vi "pumonarytesting_auto_attempt5.vi"() -> ()   [LabVIEW 2014]
uses:
  <vilib>/vision/NI_Vision_Development_Module.lvlib
  <instrlib>/KD Scientific 2XX Series/KD Scientific 2XX Series.lvlib
panel:
  in  "Start Pressure":i32=20
  in  "Number of Cycles":i32
  in  "Min Pressure":dbl
  in  "Max Pressure":dbl
  out "Status":T1
  in  "stop 2":bool
  out "Delivered Volume":dbl
  out "Units":string
  in  "Baud Rate (9600)":u32(ring)=9600 items=["300"=300, "1200"=1200, "2400"=2400, "4800"=4800, "9600"=9600]
  in  "Withdrawal Settings":T2={"Flow Rate (5)"=5.0, "Volume (10)"=10.0, "Volume Units (ml)"=enum."milliliters (ml)", "Rate Units (ml/min.)"=enum."milliliters per minute (ml/min.)"} {"Volume (10)" format="%#.3g"}
  in  "Diameter (8.75 mm)":dbl=8.75
  in  "Infusion Settings":T2={"Flow Rate (5)"=5.0, "Volume (10)"=10.0, "Volume Units (ml)"=enum."milliliters (ml)", "Rate Units (ml/min.)"=enum."milliliters per minute (ml/min.)"}
  in  "Address (0)":i32 format="%0.0f"
  in  "error in (no error)":errorcluster
  in  "VISA resource name":refnum<visa-resource-name>="COM1"
  in  "stop 4":bool
  in  "stop":bool
  out "Image":T3(plugin-control)
  out "Particle Measurements (Pixels) (Particle Analysis 1)":dbl[][](array[numeric]) format="%.2f"
  out "subarray":dbl[](array[numeric])
  out "The diameter":dbl[](array[numeric])
  in  "stop (F)":bool
  out "Data from Transducer":dynamicdata(graph) caption="Voltage from Transducer V"
  out "Voltage from pressure transducer":dbl[](array[numeric])
  out "Pressure mm Hg":dbl[](graph)
  in  "Calibration factor":dbl[](array[numeric])
  in  "Zero Error":dbl[](array[numeric])
  out "pressure mm Hg":dbl[](array[numeric])
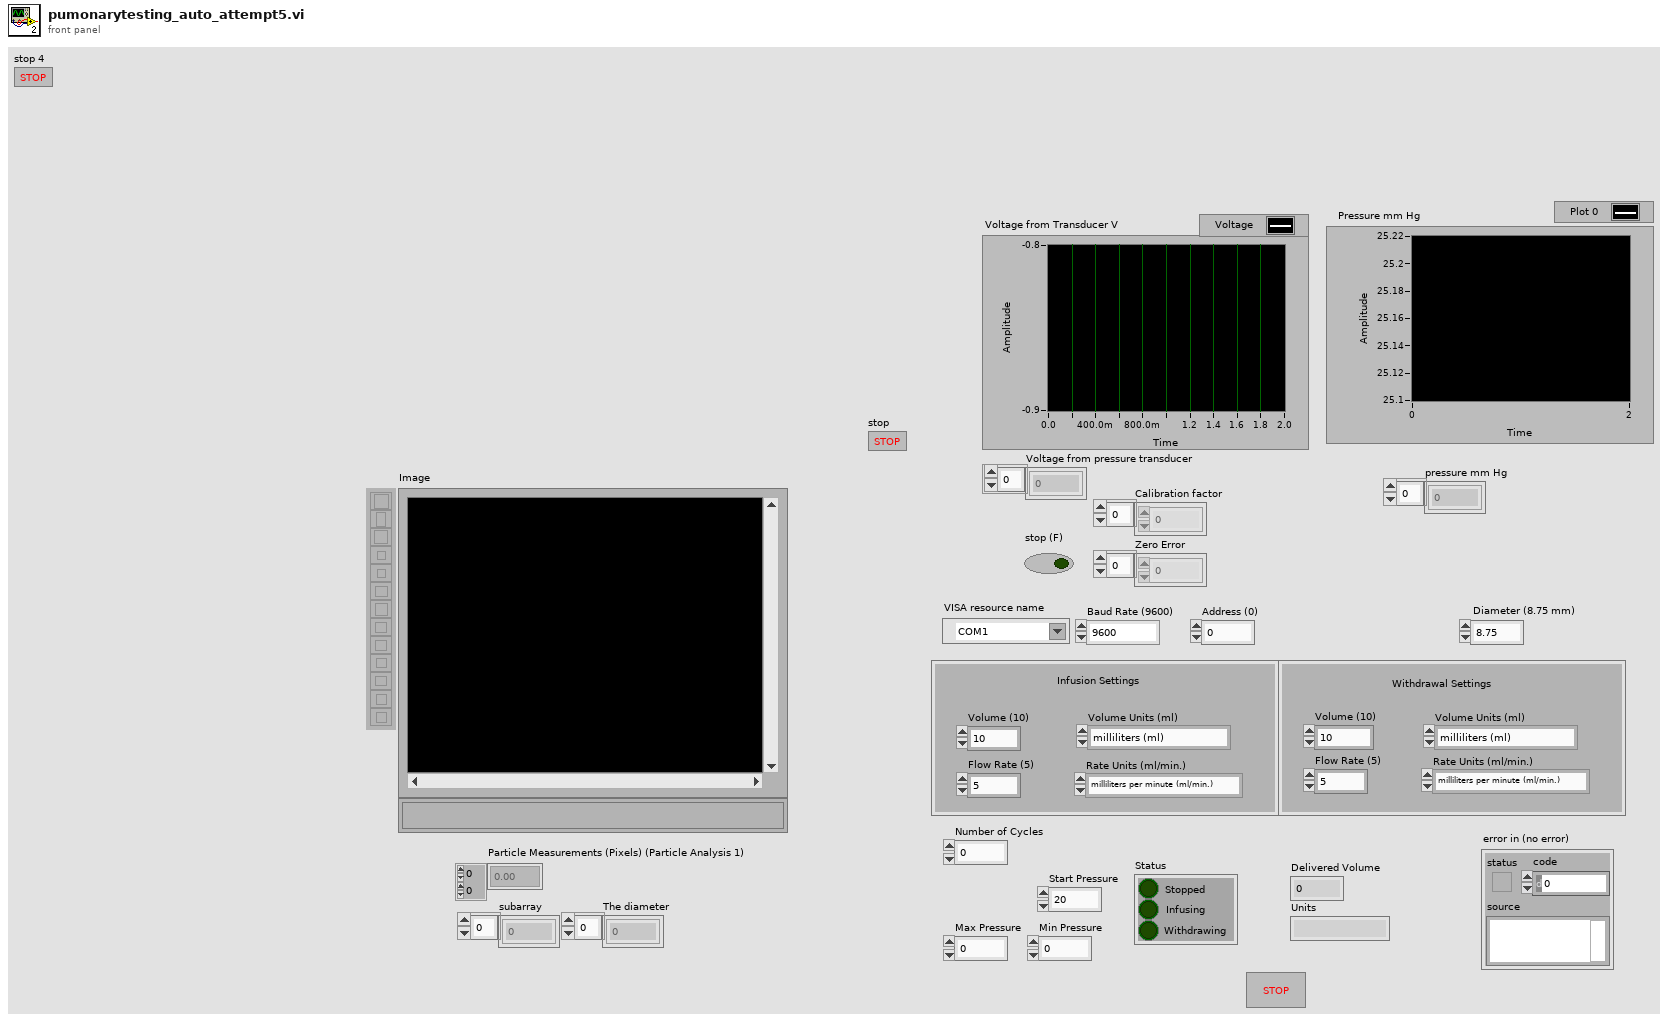
[diagram p1: front panel]
types:
  T1 = cluster{"Stopped":bool, "Infusing":bool, "Withdrawing":bool}
  T2 = cluster{"Flow Rate (5)":dbl, "Volume (10)":dbl, "Volume Units (ml)":enum16{"milliliters (ml)", "microliters (ul)"}, "Rate Units (ml/min.)":enum16{"milliliters per minute (ml/min.)", "milliliters per hour (ml/hr.)", "microliters per minute (ul/min.)", "microliters per hour (ul/hr.)"}}
  T3 = typedef "IMAQ Image.ctl" = refnum<image>
  T4 = typedef "Board Id" = u8
  T5 = typedef "ROI Descriptor" = cluster{"Global Rectangle":i32[], "Contours":cluster{"ID":enum32{"External", "Internal"}, "Type":u32, "Coordinates":i32[]}[]}
  T6 = enum16{"milliliters per minute (ml/min.)", "milliliters per hour (ml/hr.)", "microliters per minute (ul/min.)", "microliters per hour (ul/hr.)"}
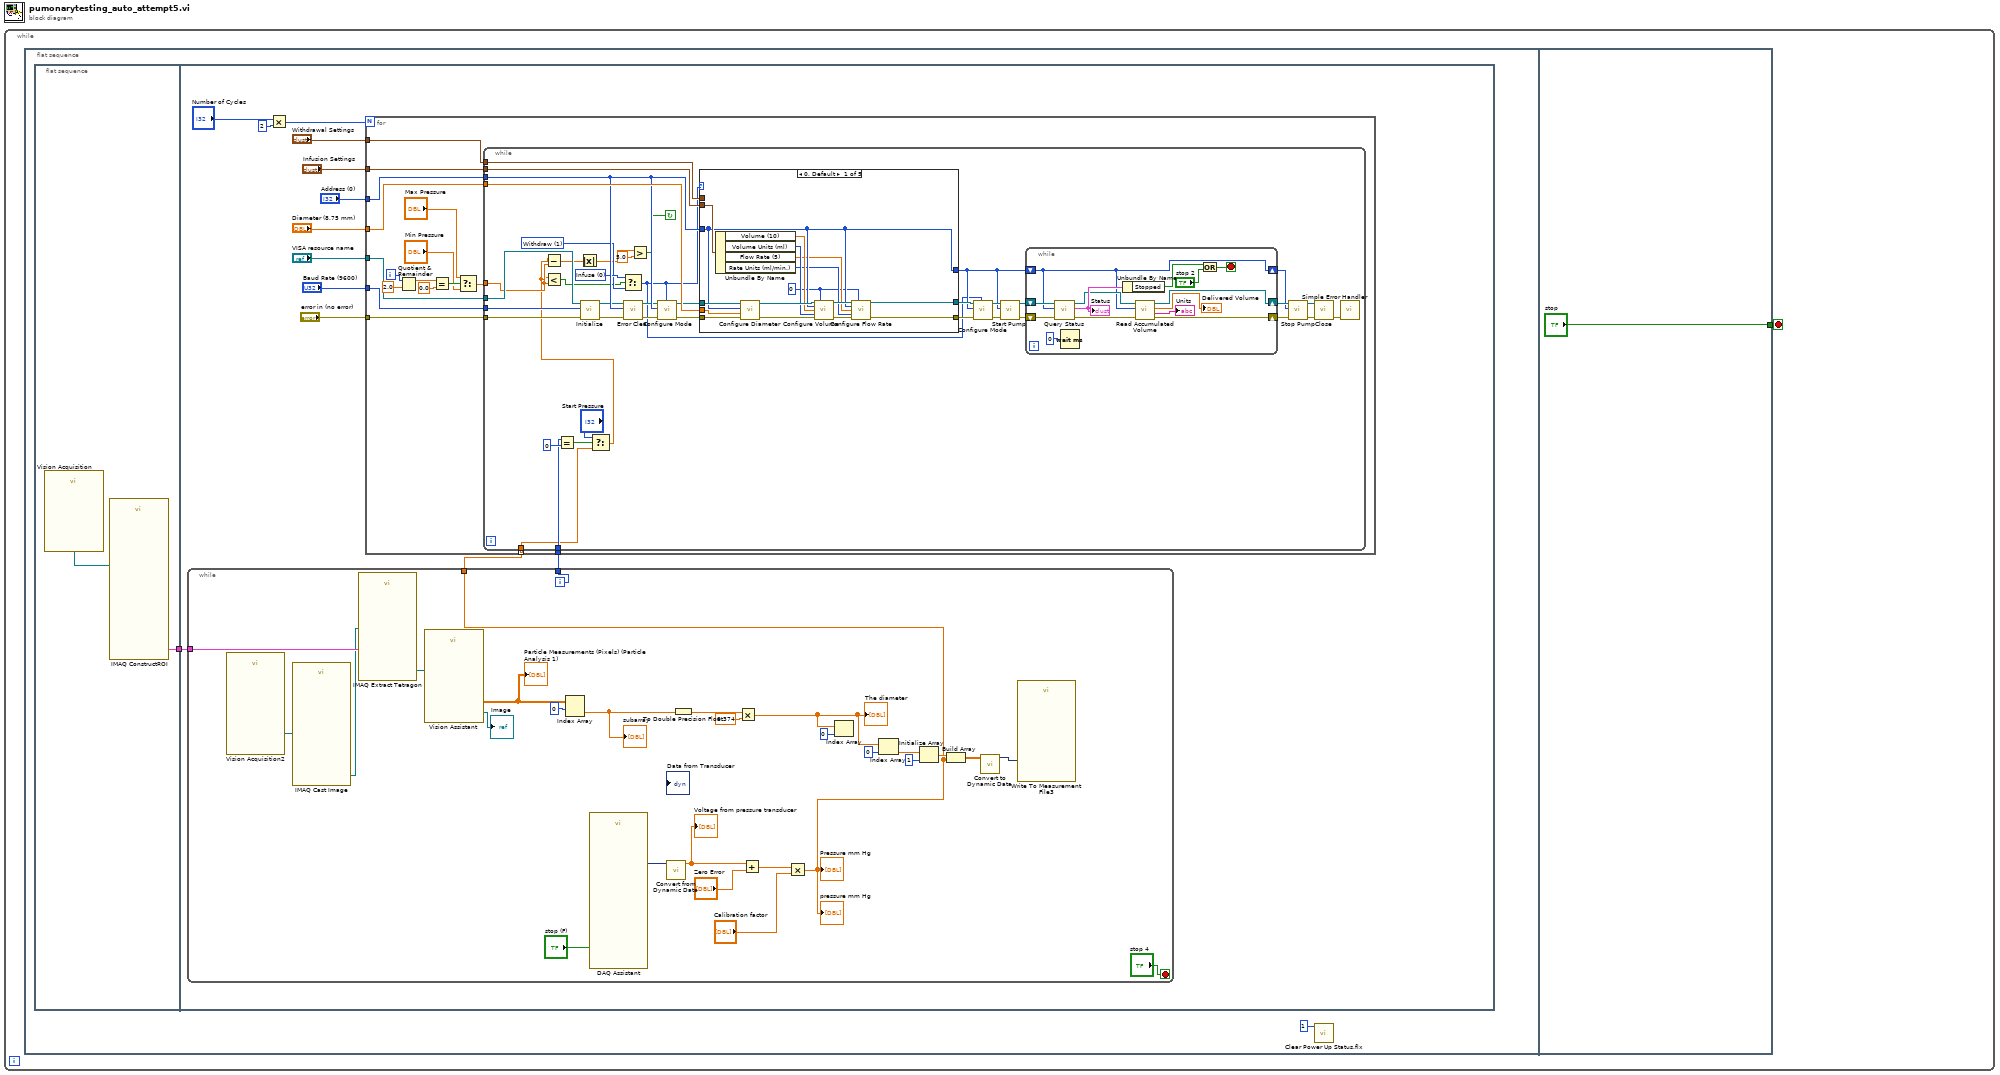
[diagram p0: block diagram]
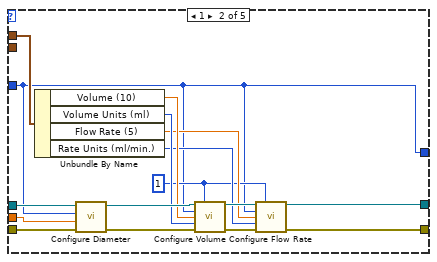
[diagram p2: hidden frame]
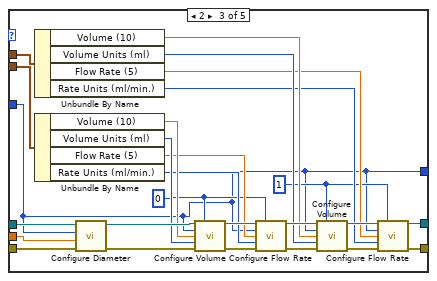
[diagram p3: hidden frame]
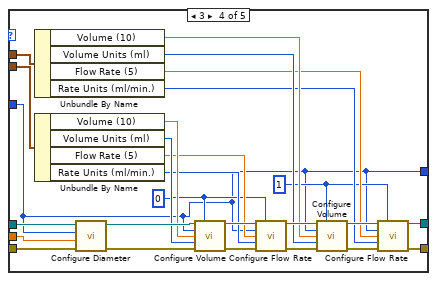
[diagram p4: hidden frame]
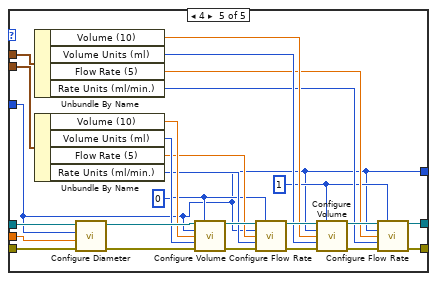
[diagram p5: hidden frame]
diagram:
  n1 = while {
    stop <- w1 stop-if-true
    n2 = flat-sequence {
      tunnel: ["stop"] -> w1
      frame #0 {
        n3 = flat-sequence {
          tunnel: [w4] -> w3
          tunnel: w3 -> [w18]
          frame #0 {
            n4 = call "Vision Acquisition"() -> ("Image Out"=w5:T3)  [unwired: 26 in, 1 out]
            n5 = call "IMAQ ConstructROI"("Image"=w5) -> ("ROI Descriptor Out"=w4:T5)  [unwired: 7 in, 3 out]
          }
          frame #1 {
            n6 = while {
              tunnel: w18 -> [w227]
              tunnel: [w202] -> w7
              tunnel: [w201] -> w6
              i -> [w201]
              stop <- "stop 4" stop-if-true
              n7 = call "Vision Acquisition2"() -> ("Image Out"=w217:T3)  [unwired: 25 in, 2 out]
              n8 = call "IMAQ Cast Image"("Image Src"=w217) -> ("Image Dst Out"=w224:T3)  [unwired: 9 in, 1 out]
              n9 = call-poly "IMAQ Extract Tetragon"("ROI Descriptor"=w227, "Image Src"=w224) -> ("Image Dst Out"=w225:T3)  [unwired: 8 in, 1 out]
              n10 = call "Vision Assistant"("Image In"=w225) -> ("Image Out"=→"Image":T3, "Particle Measurements (Pixels) (Particle Analysis 1)"=w223:dbl[][])  [unwired: 23 in, 2 out]
              "Particle Measurements (Pixels) (Particle Analysis 1)" <- w223
              n11 = Index Array(array=w223, index (row)=0) -> (element=w221:dbl[])  [unwired: 1 in]
              "subarray" <- w221
              n12 = call "DAQ Assistant"("stop (F)"="stop (F)") -> ("data"=w208:dynamicdata)  [unwired: 15 in, 3 out]
              n13 = call "Convert from Dynamic Data"("Dynamic Data Type"=w208) -> ("Array"=w205:dbl[])  [unwired: 3 in]
              "Voltage from pressure transducer" <- w205
              n14 = To Double Precision Float(number=w221) -> (double precision float=w220:dbl[])
              n15 = Multiply(x=w220, y=0.374) -> (x*y=w214:dbl[])
              "The diameter" <- w214
              n16 = Add(x=w205, y="Zero Error") -> (x+y=w207:dbl[])
              n17 = Multiply(x=w207, y="Calibration factor") -> (x*y=w202:dbl[])
              "Pressure mm Hg" <- w202
              "pressure mm Hg" <- w202
              n18 = Index Array(array=w214, index=0) -> ()  [unwired: 1 out]
              n19 = Index Array(array=w214, index=0) -> (element=w213:dbl)
              n20 = Initialize Array(w213, 1 ("dimension size")) -> (w211:dbl[])
              n21 = Build Array(w211, w202) -> (w210:dbl[][])
              n22 = call "Convert to Dynamic Data"("2D Array"=w210) -> ("Dynamic Data Type"=w209:dynamicdata)  [unwired: 3 in]
              n23 = call "Write To Measurement File3"("Signals"=w209) -> ()  [unwired: 16 in, 3 out]
            }
            n24 = Multiply(x="Number of Cycles", y=2) -> (x*y=w17:i32)
            n25 = for {
              N: w17 -> [_]
              tunnel: "VISA resource name" -> [w35]
              tunnel: "error in (no error)" -> [w34]
              tunnel: "Infusion Settings" -> [w33]
              tunnel: "Withdrawal Settings" -> [w32]
              tunnel: "Diameter (8.75 mm)" -> [w31]
              tunnel: "Baud Rate (9600)" -> [w30]
              tunnel: "Address (0)" -> [w29]
              tunnel: w7 -> [w20] mode=indexing
              tunnel: w6 -> [w19]
              i -> [w27]
              n26 = Quotient & Remainder(x=w27, y=2.0) -> (x-y*floor(x/y)=w25:dbl)  [unwired: 1 out]
              n27 = Equal?(x=w25, y=0.0) -> (x = y?=w24:bool)
              n28 = Select(t="Max Pressure", s=w24, f="Min Pressure") -> (s? t:f=w21:dbl)
              n29 = while {
                tunnel: w35 -> [w76]
                tunnel: w34 -> [w75]
                tunnel: w33 -> [w74]
                tunnel: w32 -> [w73]
                tunnel: w31 -> [w72]
                tunnel: w30 -> [w71]
                tunnel: w29 -> [w70]
                tunnel: w21 -> [w47]
                tunnel: w20 -> [w37]
                tunnel: w19 -> [w39]
                stop <- w42 continue-if-true
                w49 = u16 1 items=["Withdraw"=1]
                w50 = u16 0 items=["Infuse"] ("Mode (infuse)")
                n30 = Equal?(x=w39, y=0) -> (x = y?=w40:bool)
                n31 = call <instrlib>:"Initialize.vi"("error in (no error)"=w75, "Baud Rate (9600)"=w71, "VISA resource name"=w76) -> ("error out"=w52:errorcluster, "VISA resource name out"=w51:refnum<visa-resource-name>)  [unwired: 7 in]
                n32 = Select(t="Start Pressure", s=w40, f=w37) -> (s? t:f=w36:dbl)
                n33 = Subtract(x=w36, y=w47) -> (x-y=w46:dbl)
                n34 = Less?(x=w36, y=w47) -> (x < y?=w43:bool)
                n35 = Absolute Value(x=w46) -> (abs(x)=w45:dbl)
                n36 = Select(t=w50, s=w43, f=w49) -> (s? t:f=w48:u16)
                n37 = call <instrlib>:"Error Clear.vi"("error in (no error)"=w52, "Address (0)"=w70, "VISA resource name"=w51) -> ("error out"=w53:errorcluster, "VISA resource name out"=w54:refnum<visa-resource-name>)  [unwired: 6 in, 1 out]
                n38 = Greater?(x=w45, y=5.0) -> (0:w42:bool)
                n39 = call <instrlib>:"Configure Mode.vi"("Mode (infuse)"=w48, "error in (no error)"=w53, "Address (0)"=w70, "VISA resource name"=w54) -> ("error out"=w56:errorcluster, "VISA resource name out"=w55:refnum<visa-resource-name>)  [unwired: 6 in]
                n40 = case shown="0, Default" w48 {
                  tunnel: w74 -> [w86 _ w134 w160 w186]
                  tunnel: w73 -> [_ w108 w133 w159 w185]
                  tunnel: w55 -> [w92 w107 w132 w158 w184]
                  tunnel: w56 -> [w91 w103 w131 w157 w183]
                  tunnel: w72 -> [w85 w99 w114 w140 w166]
                  tunnel: [w84 w93 w109 w135 w161] -> w57
                  tunnel: w70 -> [w84 w93 w109 w135 w161]
                  tunnel: [w79 w104 w111 w137 w163] -> w61
                  tunnel: [w78 w100 w110 w136 w162] -> w60
                  frame 0, Default {
                    w77 = 0
                    n41 = Unbundle By Name(w86) -> ("Volume (10)"=w83:dbl, "Volume Units (ml)"=w82:enum16{"milliliters (ml)", "microliters (ul)"}, "Flow Rate (5)"=w81:dbl, "Rate Units (ml/min.)"=w80:T6)
                    n42 = call <instrlib>:"Configure Diameter.vi"("error in (no error)"=w91, "Diameter (8.75 mm)"=w85, "Address (0)"=w84, "VISA resource name"=w92) -> ("error out"=w89:errorcluster, "VISA resource name out"=w90:refnum<visa-resource-name>)  [unwired: 6 in]
                    n43 = call <instrlib>:"Configure Volume.vi"("VISA resource name"=w90, "Mode (infuse)"=w77, "Address (0)"=w84, "Volume (100)"=w83, "Units (0: milliliters)"=w82, "error in (no error)"=w89) -> ("VISA resource name out"=w88:refnum<visa-resource-name>, "error out"=w87:errorcluster)  [unwired: 8 in]
                    n44 = call <instrlib>:"Configure Flow Rate.vi"("VISA resource name"=w88, "Mode (infuse)"=w77, "Address (0)"=w84, "Flow Rate (5)"=w81, "Units (0: milliliters per minute)"=w80, "error in (no error)"=w87) -> ("VISA resource name out"=w79:refnum<visa-resource-name>, "error out"=w78:errorcluster)  [unwired: 8 in]
                  }
                  frame 1 {
                    w94 = 1
                    n45 = Unbundle By Name(w108) -> ("Volume (10)"=w98:dbl, "Volume Units (ml)"=w97:enum16{"milliliters (ml)", "microliters (ul)"}, "Flow Rate (5)"=w96:dbl, "Rate Units (ml/min.)"=w95:T6)
                    n46 = call <instrlib>:"Configure Diameter.vi"("error in (no error)"=w103, "Diameter (8.75 mm)"=w99, "Address (0)"=w93, "VISA resource name"=w107) -> ("error out"=w102:errorcluster, "VISA resource name out"=w106:refnum<visa-resource-name>)  [unwired: 6 in]
                    n47 = call <instrlib>:"Configure Volume.vi"("VISA resource name"=w106, "Mode (infuse)"=w94, "Address (0)"=w93, "Volume (100)"=w98, "Units (0: milliliters)"=w97, "error in (no error)"=w102) -> ("VISA resource name out"=w105:refnum<visa-resource-name>, "error out"=w101:errorcluster)  [unwired: 8 in]
                    n48 = call <instrlib>:"Configure Flow Rate.vi"("VISA resource name"=w105, "Mode (infuse)"=w94, "Address (0)"=w93, "Flow Rate (5)"=w96, "Units (0: milliliters per minute)"=w95, "error in (no error)"=w101) -> ("VISA resource name out"=w104:refnum<visa-resource-name>, "error out"=w100:errorcluster)  [unwired: 8 in]
                  }
                  frame 2 {
                    w112 = 1
                    w113 = 0
                    n49 = Unbundle By Name(w133) -> ("Volume (10)"=w118:dbl, "Volume Units (ml)"=w117:enum16{"milliliters (ml)", "microliters (ul)"}, "Flow Rate (5)"=w116:dbl, "Rate Units (ml/min.)"=w115:T6)
                    n50 = Unbundle By Name(w134) -> ("Volume (10)"=w122:dbl, "Volume Units (ml)"=w121:enum16{"milliliters (ml)", "microliters (ul)"}, "Flow Rate (5)"=w120:dbl, "Rate Units (ml/min.)"=w119:T6)
                    n51 = call <instrlib>:"Configure Diameter.vi"("error in (no error)"=w131, "Diameter (8.75 mm)"=w114, "Address (0)"=w109, "VISA resource name"=w132) -> ("error out"=w126:errorcluster, "VISA resource name out"=w130:refnum<visa-resource-name>)  [unwired: 6 in]
                    n52 = call <instrlib>:"Configure Volume.vi"("VISA resource name"=w130, "Mode (infuse)"=w113, "Address (0)"=w109, "Volume (100)"=w122, "Units (0: milliliters)"=w121, "error in (no error)"=w126) -> ("VISA resource name out"=w129:refnum<visa-resource-name>, "error out"=w125:errorcluster)  [unwired: 8 in]
                    n53 = call <instrlib>:"Configure Flow Rate.vi"("VISA resource name"=w129, "Mode (infuse)"=w113, "Address (0)"=w109, "Flow Rate (5)"=w120, "Units (0: milliliters per minute)"=w119, "error in (no error)"=w125) -> ("VISA resource name out"=w128:refnum<visa-resource-name>, "error out"=w124:errorcluster)  [unwired: 8 in]
                    n54 = call <instrlib>:"Configure Volume.vi"("VISA resource name"=w128, "Mode (infuse)"=w112, "Address (0)"=w109, "Volume (100)"=w118, "Units (0: milliliters)"=w117, "error in (no error)"=w124) -> ("VISA resource name out"=w127:refnum<visa-resource-name>, "error out"=w123:errorcluster)  [unwired: 8 in]
                    n55 = call <instrlib>:"Configure Flow Rate.vi"("VISA resource name"=w127, "Mode (infuse)"=w112, "Address (0)"=w109, "Flow Rate (5)"=w116, "Units (0: milliliters per minute)"=w115, "error in (no error)"=w123) -> ("VISA resource name out"=w111:refnum<visa-resource-name>, "error out"=w110:errorcluster)  [unwired: 8 in]
                  }
                  frame 3 {
                    w138 = 1
                    w139 = 0
                    n56 = Unbundle By Name(w159) -> ("Volume (10)"=w144:dbl, "Volume Units (ml)"=w143:enum16{"milliliters (ml)", "microliters (ul)"}, "Flow Rate (5)"=w142:dbl, "Rate Units (ml/min.)"=w141:T6)
                    n57 = Unbundle By Name(w160) -> ("Volume (10)"=w148:dbl, "Volume Units (ml)"=w147:enum16{"milliliters (ml)", "microliters (ul)"}, "Flow Rate (5)"=w146:dbl, "Rate Units (ml/min.)"=w145:T6)
                    n58 = call <instrlib>:"Configure Diameter.vi"("error in (no error)"=w157, "Diameter (8.75 mm)"=w140, "Address (0)"=w135, "VISA resource name"=w158) -> ("error out"=w152:errorcluster, "VISA resource name out"=w156:refnum<visa-resource-name>)  [unwired: 6 in]
                    n59 = call <instrlib>:"Configure Volume.vi"("VISA resource name"=w156, "Mode (infuse)"=w139, "Address (0)"=w135, "Volume (100)"=w148, "Units (0: milliliters)"=w147, "error in (no error)"=w152) -> ("VISA resource name out"=w155:refnum<visa-resource-name>, "error out"=w151:errorcluster)  [unwired: 8 in]
                    n60 = call <instrlib>:"Configure Flow Rate.vi"("VISA resource name"=w155, "Mode (infuse)"=w139, "Address (0)"=w135, "Flow Rate (5)"=w146, "Units (0: milliliters per minute)"=w145, "error in (no error)"=w151) -> ("VISA resource name out"=w154:refnum<visa-resource-name>, "error out"=w150:errorcluster)  [unwired: 8 in]
                    n61 = call <instrlib>:"Configure Volume.vi"("VISA resource name"=w154, "Mode (infuse)"=w138, "Address (0)"=w135, "Volume (100)"=w144, "Units (0: milliliters)"=w143, "error in (no error)"=w150) -> ("VISA resource name out"=w153:refnum<visa-resource-name>, "error out"=w149:errorcluster)  [unwired: 8 in]
                    n62 = call <instrlib>:"Configure Flow Rate.vi"("VISA resource name"=w153, "Mode (infuse)"=w138, "Address (0)"=w135, "Flow Rate (5)"=w142, "Units (0: milliliters per minute)"=w141, "error in (no error)"=w149) -> ("VISA resource name out"=w137:refnum<visa-resource-name>, "error out"=w136:errorcluster)  [unwired: 8 in]
                  }
                  frame 4 {
                    w164 = 1
                    w165 = 0
                    n63 = Unbundle By Name(w185) -> ("Volume (10)"=w170:dbl, "Volume Units (ml)"=w169:enum16{"milliliters (ml)", "microliters (ul)"}, "Flow Rate (5)"=w168:dbl, "Rate Units (ml/min.)"=w167:T6)
                    n64 = Unbundle By Name(w186) -> ("Volume (10)"=w174:dbl, "Volume Units (ml)"=w173:enum16{"milliliters (ml)", "microliters (ul)"}, "Flow Rate (5)"=w172:dbl, "Rate Units (ml/min.)"=w171:T6)
                    n65 = call <instrlib>:"Configure Diameter.vi"("error in (no error)"=w183, "Diameter (8.75 mm)"=w166, "Address (0)"=w161, "VISA resource name"=w184) -> ("error out"=w178:errorcluster, "VISA resource name out"=w182:refnum<visa-resource-name>)  [unwired: 6 in]
                    n66 = call <instrlib>:"Configure Volume.vi"("VISA resource name"=w182, "Mode (infuse)"=w165, "Address (0)"=w161, "Volume (100)"=w174, "Units (0: milliliters)"=w173, "error in (no error)"=w178) -> ("VISA resource name out"=w181:refnum<visa-resource-name>, "error out"=w177:errorcluster)  [unwired: 8 in]
                    n67 = call <instrlib>:"Configure Flow Rate.vi"("VISA resource name"=w181, "Mode (infuse)"=w165, "Address (0)"=w161, "Flow Rate (5)"=w172, "Units (0: milliliters per minute)"=w171, "error in (no error)"=w177) -> ("VISA resource name out"=w180:refnum<visa-resource-name>, "error out"=w176:errorcluster)  [unwired: 8 in]
                    n68 = call <instrlib>:"Configure Volume.vi"("VISA resource name"=w180, "Mode (infuse)"=w164, "Address (0)"=w161, "Volume (100)"=w170, "Units (0: milliliters)"=w169, "error in (no error)"=w176) -> ("VISA resource name out"=w179:refnum<visa-resource-name>, "error out"=w175:errorcluster)  [unwired: 8 in]
                    n69 = call <instrlib>:"Configure Flow Rate.vi"("VISA resource name"=w179, "Mode (infuse)"=w164, "Address (0)"=w161, "Flow Rate (5)"=w168, "Units (0: milliliters per minute)"=w167, "error in (no error)"=w175) -> ("VISA resource name out"=w163:refnum<visa-resource-name>, "error out"=w162:errorcluster)  [unwired: 8 in]
                  }
                }
                n70 = call <instrlib>:"Configure Mode.vi"("Mode (infuse)"=w48, "error in (no error)"=w60, "Address (0)"=w57, "VISA resource name"=w61) -> ("error out"=w58:errorcluster, "VISA resource name out"=w59:refnum<visa-resource-name>)  [unwired: 6 in]
                n71 = call <instrlib>:"Start Pump.vi"("error in (no error)"=w58, "Address (0)"=w57, "VISA resource name"=w59) -> ("error out"=w68:errorcluster, "VISA resource name out"=w69:refnum<visa-resource-name>)  [unwired: 7 in]
                n72 = while {
                  shift-right: [w189] -> w65
                  shift-left: w57 -> [w189]
                  shift-right: [w191] -> w67
                  shift-left: w69 -> [w197]
                  shift-right: [w190] -> w66
                  shift-left: w68 -> [w198]
                  stop <- w195 stop-if-true
                  n73 = call <instrlib>:"Query Status.vi"("error in (no error)"=w198, "Address (0)"=w189, "VISA resource name"=w197) -> ("error out"=w200:errorcluster, "Status"=w196:T1, "VISA resource name out"=w192:refnum<visa-resource-name>)  [unwired: 6 in]
                  "Status" <- w196
                  n74 = Wait (ms)(milliseconds to wait=u32 0) -> ()  [unwired: 1 out]
                  n75 = Unbundle By Name(w196) -> ("Stopped"=w194:bool)
                  n76 = call <instrlib>:"Read Accumulated Volume.vi"("error in (no error)"=w200, "Address (0)"=w189, "VISA resource name"=w192) -> ("error out"=w190:errorcluster, "Units"=→"Units":string, "Delivered Volume"=→"Delivered Volume":dbl, "VISA resource name out"=w191:refnum<visa-resource-name>)  [unwired: 5 in]
                  n77 = Or(x=w194, y="stop 2") -> (x .or. y?=w195:bool)
                }
                n78 = call <instrlib>:"Stop Pump.vi"("error in (no error)"=w66, "Address (0)"=w65, "VISA resource name"=w67) -> ("error out"=w63:errorcluster, "VISA resource name out"=w62:refnum<visa-resource-name>)  [unwired: 7 in]
                n79 = call <instrlib>:"Close.vi"("error in (no error)"=w63, "VISA resource name"=w62) -> ("error out"=w64:errorcluster)  [unwired: 9 in]
                n80 = call <vilib>:"Simple Error Handler.vi"("error in (no error)"=w64) -> ()  [unwired: 4 in, 5 out]
              }
            }
          }
        }
        n81 = call <vilib>:"Clear Power Up Status.flx"("Board ID"=T4 1) -> ()  [unwired: 6 in, 2 out]
      }
      frame #1 {
      }
    }
  }
